vi "Shutdown.vi"(11 "Network Session in":refnum<class "Network Session Handler.lvclass">) -> ()   [LabVIEW 2017, in "Network Interface.lvlib" / "Network Session Handler.lvclass"]
uses:
  <vilib>/gpm_packages/@cs/Network-sink/Source/Network Interface/Network Session Handler/Network Session Handler.lvclass
  <vilib>/gpm_packages/@cs/Network-sink/Source/Network Interface/Connection Handler/Message Names ENUM.ctl
  <vilib>/gpm_packages/@cs/event-logger/Source/Composed Log/Types/Log Level.ctl
  <vilib>/gpm_packages/@cs/Network-sink/Source/Network Interface/Network Session Handler/Network Session Handler.lvclass/Network Session Handler.ctl
  <vilib>/gpm_packages/@cs/event-logger/Source/Composed Log/LoggerReference/LoggerReference.lvclass/LoggerReference.ctl
  <vilib>/gpm_packages/@cs/Network-sink/Source/Network Interface/Message Queue/Message Queue.lvclass/Message Queue.ctl
  <vilib>/gpm_packages/@cs/Network-sink/Source/Network Interface/Connection Handler/Synchronous Write Request.ctl
  247c51b6-9884-41c7-850d-0467b4e5cca4.vi
  <vilib>/gpm_packages/@cs/Network-sink/Source/Network Interface/Message Queue/Protected Enqueue.vi
  <vilib>/gpm_packages/@cs/event-logger/Source/Composed Log/LoggerReference/Log.vi
  <vilib>/gpm_packages/@cs/event-logger/Source/Composed Log/LoggerReference/Get Valid Event Time.vi
  <vilib>/gpm_packages/@cs/event-logger/Source/Composed Log/LoggerReference/Remove Stale Logs.vi
  <vilib>/Utility/error.llb/Error Cluster From Error Code.vi
  <vilib>/ErrorRing/Error Ring.xnode
  <vilib>/gpm_packages/@cs/Network-sink/Source/Network Interface/IConnectionFactory/IConnectionFactory.lvclass
  <vilib>/gpm_packages/@cs/Network-sink/Source/Network Interface/Message Queue/Message Queue.lvclass
  <vilib>/gpm_packages/@cs/Network-sink/Source/Network Interface/Connection Handler/Connection Handler.lvclass
  <vilib>/gpm_packages/@cs/event-logger/Source/Composed Log/Composed Log.lvlib
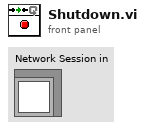
[diagram p1: front panel]
types:
  T1 = typedef "Composed Log.lvlib/Log Level.ctl" = enum16{"Debug", "Info", "Warning", "Error", "Critical"}
  T2 = typedef "Network Interface.lvlib/Connection Handler.lvclass/Message Names ENUM.ctl" = enum16{"Transmit Message", "Stop"}
  T3 = typedef "Network Interface.lvlib/Message Queue.lvclass/Message Cluster.ctl" = cluster{"Msg":string, "Data":variant}
  T4 = typedef "Network Interface.lvlib/Network Session Handler.lvclass/Connection Handler.ctl" = cluster{"ID":string, "Handler Queue":refnum<class "Message Queue.lvclass">}
  T5 = typedef "Network Interface.lvlib/Connection Handler.lvclass/Synchronous Write Request.ctl" = cluster{"Data To Write":string, "Return Queue":refnum<queue>}
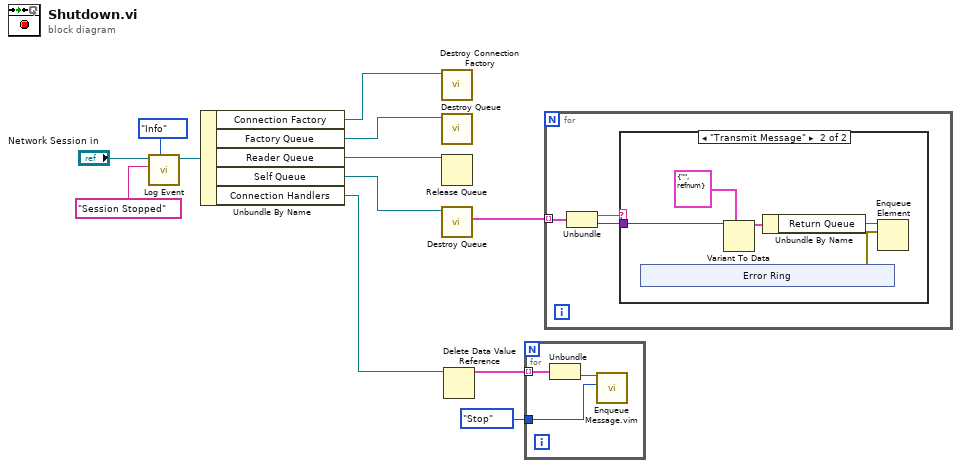
[diagram p0: block diagram]
diagram:
  n1 = call <vilib>:"Log Event.vi"("Event Level"=Log_Level."Info", "Event"="Session Stopped", "Network Session Handler in"="Network Session in") -> ("Network Session Handler out"=w3:refnum<class "Network Session Handler.lvclass">)  [unwired: 7 in, 1 out]
  n2 = Unbundle By Name(w3) -> ("Connection Factory"=w12:refnum<class "IConnectionFactory.lvclass">, "Factory Queue"=w11:refnum<class "Message Queue.lvclass">, "Reader Queue"=w9:refnum<queue>, "Self Queue"=w10:refnum<class "Message Queue.lvclass">, "Connection Handlers"=w8:refnum<data-value>)
  n3 = call-dynamic "Destroy Connection Factory.vi"("IConnectionFactory in"=w12) -> ()  [unwired: 10 in, 1 out]
  n4 = call <vilib>:"Destroy Queue.vi"("Message Queue in"=w11) -> ()  [unwired: 8 in, 3 out]
  n5 = Release Queue(queue=w9) -> ()  [unwired: 2 in, 3 out]
  n6 = call <vilib>:"Destroy Queue.vi"("Message Queue in"=w10) -> ("Remaining Elements"=w5:T3[])  [unwired: 8 in, 2 out]
  n7 = Delete Data Value Reference(data value reference=w8) -> (data value=w7:T4[])  [unwired: 1 in, 1 out]
  n8 = for {
    tunnel: w7 -> [w14] mode=indexing
    tunnel: Message_Names_ENUM."Stop" ("Messages") -> [w15]
    n9 = Unbundle(w14) -> ("Handler Queue"=w13:refnum<class "Message Queue.lvclass">)  [unwired: 1 out]
    n10 = call "Enqueue Message.vim"("Msg"=w15, "Message Queue in"=w13) -> ()  [unwired: 8 in, 2 out]
  }
  n11 = for {
    tunnel: w5 -> [w18] mode=indexing
    n12 = Unbundle(w18) -> ("Msg"=w17:string, "Data"=w16:variant)
    n13 = case shown="\"Transmit Message\"" w17 {
      tunnel: w16 -> [_ w22]
      frame "False", Default {
      }
      frame "Transmit Message" {
        n14 = xnode "Error Ring"() -> ("error out"=w19:errorcluster)
        n15 = Variant To Data(type=T5 {"Data To Write"="", "Return Queue"=refnum} ("Write Request"), Variant=w22) -> (data=w21:T5)  [unwired: 1 in, 1 out]
        n16 = Unbundle By Name(w21) -> ("Return Queue"=w20:refnum<queue>)
        n17 = Enqueue Element(queue=w20, element=w19) -> ()  [unwired: 2 in, 3 out]
      }
    }
  }
